vi "Fetch 5034B.vi"(8 "error in (no error)":errorcluster, 9 "MaxTime (10000ms)":u32=10000, 10 "Ch (1=Ch1)":u16(ring) items=["None", "Channel1", "Channel2", "Channel3", "Channel4", "Math1", "Math2", "Math3", "Math3", "Reference1", "Reference2", "Reference3", "Reference4"], 11 "VISA resource name":refnum<visa-resource-name>) -> (0 "error out":errorcluster, 1 "Data Cluster":cluster{"Y":dbl[], "t0":dbl, "dt":dbl}, 2 "Waveform Data":waveform(dbl)(graph)={"t0"=timestamp(3.694502999999883e-07 s since 1904-01-01), "dt"=5e-07, "Y"=array[10000 elements]}, 3 "VISA ResNameOut":refnum<visa-resource-name>)   [LabVIEW 2012]
doc: "Returns the waveform that an oscilloscope acquires for a channel you specify. An acquisition that you initiate before calling this VI generates the waveform.\n\nYou first enable channels with the tkdpo7k Configure Channel VI. Then you use the tkdpo7k Initiate VI to start an acquisition on the enabled channels. An oscilloscope concurrently acquires waveforms for these channels. You must call the tkdpo7k Fetch Waveform VI separately to obtain waveforms for each enabled channel. However, you also can call the tkdpo7k Read Waveform VI instead of using the above low-level VIs.\n\n<B>Note:</B> Use the tkdpo7k Fetch Waveform VI only with other low-level VIs, such as the tkdpo7k Initiate VI, the tkdpo7k Abort VI, and the tkdpo7k Fetch Waveform Measurement VI. High-level VIs such as the tkdpo7k Read Waveform VI automatically incorporate the functions of the tkdpo7k Initiate VI and the tkdpo7kFetch Waveform VI. The tkdpo7k Fetch Waveform VI does not check the status of an instrument."
panel:
  out "Data5064":dbl[](array[numeric])
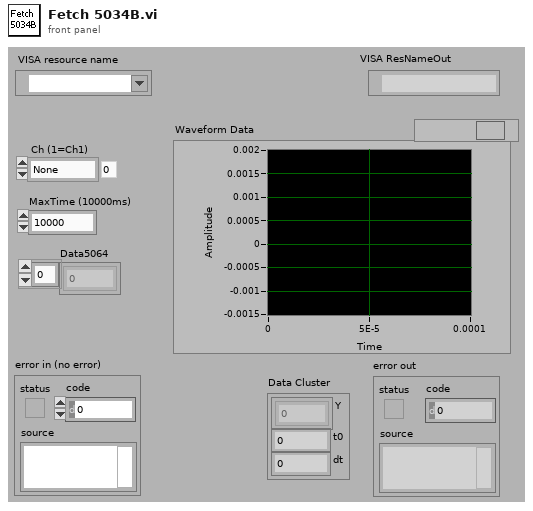
[diagram p1: front panel]
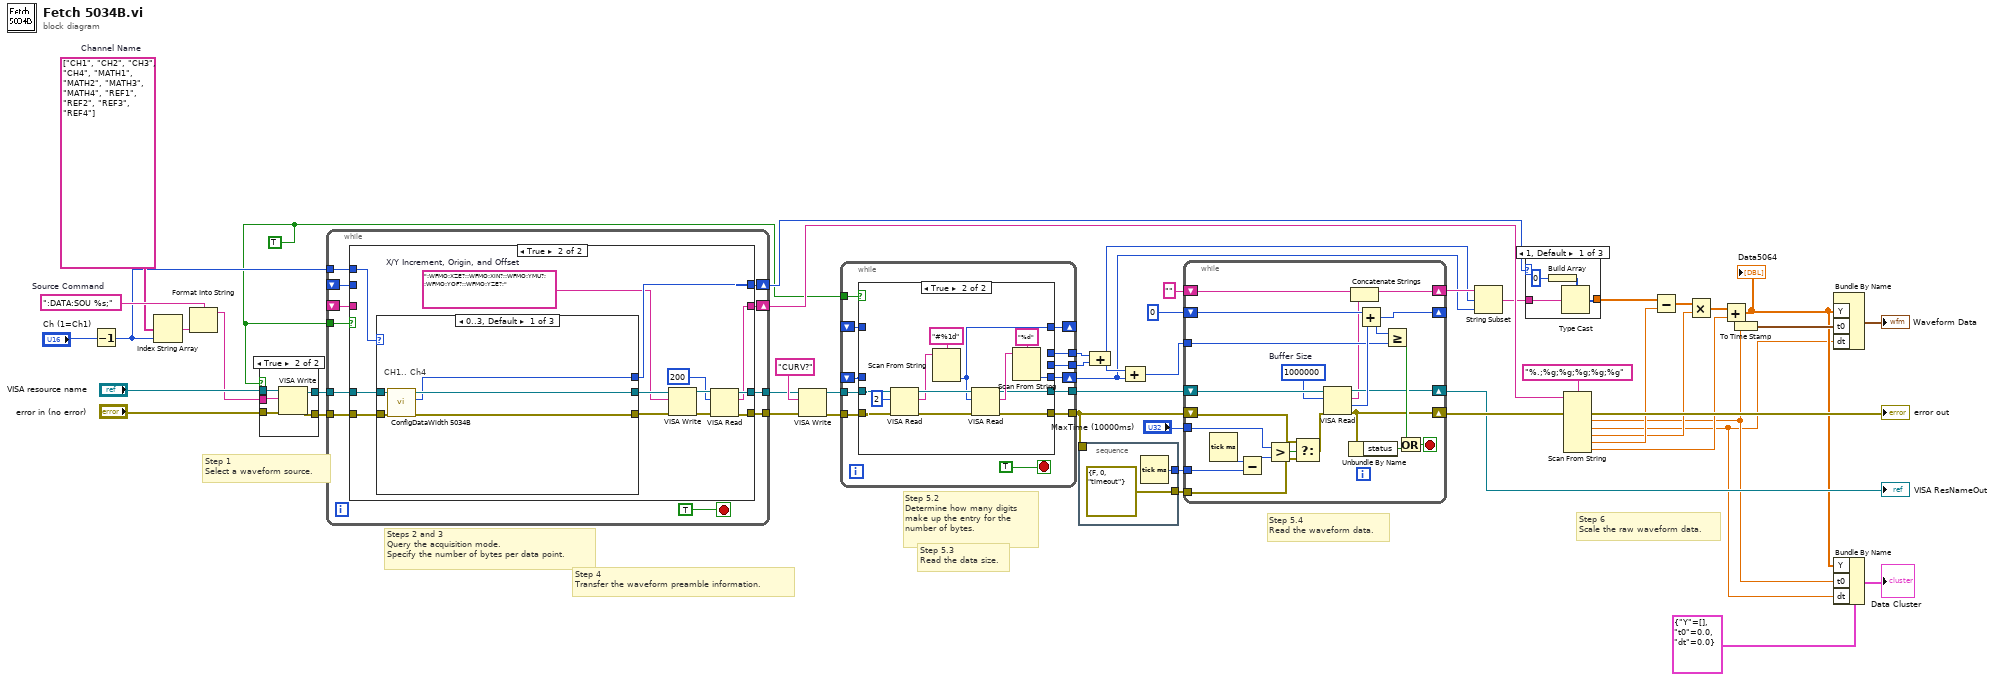
[diagram p0: block diagram]
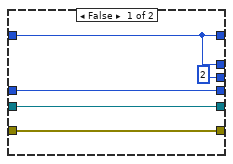
[diagram p3: hidden frame]
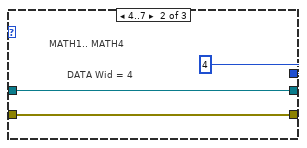
[diagram p5: hidden frame]
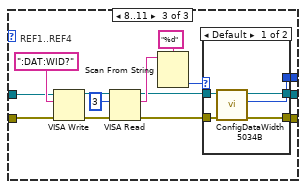
[diagram p6: hidden frame]
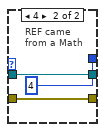
[diagram p7: hidden frame]
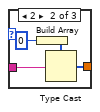
[diagram p8: hidden frame]
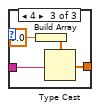
[diagram p9: hidden frame]
diagram:
  w6 = TRUE
  w37 = string[] ["CH1", "CH2", "CH3", "CH4", "MATH1", "MATH2", "MATH3", "MATH4", "REF1", "REF2", "REF3", "REF4"]  # Channel Name
  w49 = ":DATA:SOU %s;"  # Source Command
  # "Step 1       \nSelect a waveform source."
  # "Steps 2 and 3\nQuery the acquisition mode. \nSpecify the number of bytes per data point."
  # "Step 6    \nScale the raw waveform data."
  # "Step 5.4   \nRead the waveform data."
  # "Step 5.3      \nRead the data size."
  # "Step 5.2      \nDetermine how many digits\nmake up the entry for the \nnumber of bytes."
  # "Step 4\nTransfer the waveform preamble information."
  n1 = Decrement(x="Ch (1=Ch1)") -> (x-1=w7:u16)
  n2 = Index String Array(1:w7, 2:w37) -> (0:w48:string)  [unwired: 1 in]
  n3 = Format Into String(format string=w49, w48) -> (resulting string=w34:string)  [unwired: 2 in, 1 out]
  n4 = case shown="True" w6 {
    tunnel: "VISA resource name" -> [w51 w56]
    tunnel: "error in (no error)" -> [w50 w55]
    tunnel: w34 -> [_ w54]
    tunnel: [w51 w53] -> w31
    tunnel: [w50 w52] -> w30
    frame False {
    }
    frame True {
      n5 = VISA Write(VISA resource name=w56, write buffer=w54, error in (no error)=w55) -> (VISA resource name out=w53:refnum<visa-resource-name>, error out=w52:errorcluster)  [unwired: 1 out]
    }
  }
  n6 = while {
    tunnel: w7 -> [w67]
    tunnel: w31 -> [w66]
    tunnel: w30 -> [w65]
    tunnel: [w63] -> w21
    tunnel: [w62] -> w20
    tunnel: w6 -> [w61]
    shift-right: [w64] -> w23
    shift-left: _ -> [w59]
    shift-right: [w58] -> w22
    shift-left: _ -> [w57]
    stop <- TRUE stop-if-true
    n7 = case shown="True" w61 {
      tunnel: w67 -> [_ w84]
      tunnel: w66 -> [w71 w83]
      tunnel: w65 -> [w70 w82]
      tunnel: [w69 w81] -> w64
      tunnel: [w71 w75] -> w63
      tunnel: [w70 w74] -> w62
      tunnel: w59 -> [w69 _]
      tunnel: [w68 w72] -> w58
      tunnel: w57 -> [w68 _]
      frame False {
      }
      frame True {
        w73 = ":WFMO:XZE?;:WFMO:XIN?;:WFMO:YMU?;:WFMO:YOF?;:WFMO:YZE?;"  # X/Y Increment, Origin, and Offset
        n8 = case shown="0..3, Default" w84 {
          tunnel: w83 -> [w89 w92 w101]
          tunnel: w82 -> [w88 w91 w102]
          tunnel: [w87 w92 w95] -> w77
          tunnel: [w86 w91 w94] -> w76
          tunnel: [w85 u32 4 ("byte count") w93] -> w81
          frame 0..3, Default {
            # "CH1.. Ch4"
            n9 = call "ConfigDataWidth 5034B.vi"("error in (no error)"=w88, "VISA resource name"=w89) -> ("error out"=w86:errorcluster, "Width"=w85:i32, "VISA res name out"=w87:refnum<visa-resource-name>)  [unwired: 7 in]
          }
          frame 4..7 {
            # "DATA Wid = 4"
            # "MATH1.. MATH4"
          }
          frame 8..11 {
            # "REF1..REF4"
            n10 = VISA Write(VISA resource name=w101, write buffer=":DAT:WID?", error in (no error)=w102) -> (VISA resource name out=w106:refnum<visa-resource-name>, error out=w105:errorcluster)  [unwired: 1 out]
            n11 = VISA Read(VISA resource name=w106, byte count=u32 3, error in (no error)=w105) -> (VISA resource name out=w97:refnum<visa-resource-name>, read buffer=w100:string, error out=w96:errorcluster)  [unwired: 1 out]
            n12 = Scan From String(format string="%d", input string=w100) -> (output 1=w98:i32)  [unwired: 3 in, 3 out]
            n13 = case shown="Default" w98 {
              tunnel: w97 -> [w111 w114]
              tunnel: w96 -> [w110 w113]
              tunnel: [w109 w114] -> w95
              tunnel: [w108 w113] -> w94
              tunnel: [w107 u32 4 ("byte count")] -> w93
              frame Default {
                n14 = call "ConfigDataWidth 5034B.vi"("error in (no error)"=w110, "VISA resource name"=w111) -> ("error out"=w108:errorcluster, "Width"=w107:i32, "VISA res name out"=w109:refnum<visa-resource-name>)  [unwired: 7 in]
              }
              frame 4 {
                # "REF came\nfrom a Math"
              }
            }
          }
        }
        n15 = VISA Write(VISA resource name=w77, write buffer=w73, error in (no error)=w76) -> (VISA resource name out=w79:refnum<visa-resource-name>, error out=w80:errorcluster)  [unwired: 1 out]
        n16 = VISA Read(VISA resource name=w79, byte count=u32 200, error in (no error)=w80) -> (VISA resource name out=w75:refnum<visa-resource-name>, read buffer=w72:string, error out=w74:errorcluster)  [unwired: 1 out]
      }
    }
  }
  n17 = VISA Write(VISA resource name=w21, write buffer="CURV?" ("Curve Command"), error in (no error)=w20) -> (VISA resource name out=w29:refnum<visa-resource-name>, error out=w46:errorcluster)  [unwired: 1 out]
  n18 = while {
    tunnel: w46 -> [w126]
    tunnel: w29 -> [w125]
    tunnel: [w124] -> w28
    tunnel: [w123] -> w9
    tunnel: w6 -> [w122]
    shift-right: [w120] -> w11
    shift-left: _ -> [w119]
    shift-right: [w116] -> _
    shift-left: _ -> [w118]
    tunnel: [w117] -> w14
    tunnel: [w115] -> w13
    stop <- TRUE stop-if-true
    n19 = case shown="True" w122 {
      tunnel: w126 -> [w129 w144]
      tunnel: w125 -> [w130 w137]
      tunnel: [w130 w136] -> w124
      tunnel: [w129 w135] -> w123
      tunnel: [w131 w133] -> w120
      tunnel: w119 -> [w131 _]
      tunnel: [w127 w132] -> w116
      tunnel: w118 -> [w127 _]
      tunnel: [u32 2 ("byte count") _] -> w117
      tunnel: [w127 _] -> w115
      frame False {
      }
      frame True {
        n20 = VISA Read(VISA resource name=w137, byte count=u32 2, error in (no error)=w144) -> (VISA resource name out=w142:refnum<visa-resource-name>, read buffer=w140:string, error out=w141:errorcluster)  [unwired: 1 out]
        n21 = Scan From String(format string="#%1d", input string=w140) -> (output 1=w132:i32)  [unwired: 3 in, 3 out]
        n22 = VISA Read(VISA resource name=w142, byte count=w132, error in (no error)=w141) -> (VISA resource name out=w136:refnum<visa-resource-name>, read buffer=w138:string, error out=w135:errorcluster)  [unwired: 1 out]
        n23 = Scan From String(format string="%d", input string=w138) -> (output 1=w133:i32)  [unwired: 3 in, 3 out]
      }
    }
  }
  n24 = stacked-sequence {
    tunnel: [w146] -> w25
    tunnel: [errorcluster {"status"=FALSE, "code"=0, "source"="timeout"} ("error out")] -> w19
    tunnel: w9 -> [_]
    frame #0 {
      n25 = Tick Count (ms)() -> (millisecond timer value=w146:u32)
    }
  }
  n26 = Compound Arithmetic op=ADD(w13, w14) -> (w12:u32)
  n27 = Compound Arithmetic op=ADD(w12, w11) -> (w15:u32)
  n28 = while {
    shift-right: [w151] -> w43
    shift-left: w28 -> [w168]
    shift-right: [w147] -> w45
    shift-left: w9 -> [w155]
    shift-right: [w148] -> w16
    shift-left: "" -> [w150]
    tunnel: w15 -> [w153]
    shift-right: [w165] -> _
    shift-left: u32 0 -> [w166]
    tunnel: w25 -> [w163]
    tunnel: "MaxTime (10000ms)" -> [w162]
    tunnel: w19 -> [w160]
    stop <- w158 stop-if-true
    w152 = 1000000  # Buffer Size
    n29 = Tick Count (ms)() -> (millisecond timer value=w164:u32)
    n30 = Subtract(x=w164, y=w163) -> (x-y=w161:u32)
    n31 = Greater?(x=w162, y=w161) -> (0:w154:bool)
    n32 = Select(t=w155, s=w154, f=w160) -> (s? t:f=w157:errorcluster)
    n33 = VISA Read(VISA resource name=w168, byte count=w152, error in (no error)=w157) -> (VISA resource name out=w151:refnum<visa-resource-name>, read buffer=w149:string, return count=w167:u32, error out=w147:errorcluster)
    n34 = Unbundle By Name(w147) -> ("status"=w156:bool)
    n35 = Concatenate Strings(w150, w149) -> (w148:string)
    n36 = Add(x=w166, y=w167) -> (x+y=w165:u32)
    n37 = Greater Or Equal?(x=w165, y=w153) -> (x >= y?=w159:bool)
    n38 = Or(x=w159, y=w156) -> (x .or. y?=w158:bool)
  }
  "VISA ResNameOut" <- w43
  n39 = String Subset(string=w16, offset (0)=w12, length (rest)=w11) -> (substring=w10:string)
  n40 = case shown="1, Default" w23 {
    tunnel: w10 -> [w170 w174 w178]
    tunnel: [w169 w173 w177] -> w32
    frame 1, Default {
      n41 = Build Array(i8 0) -> (w171:i8[])
      n42 = Type Cast(type=w171, x=w170) -> (*(type *) &x=w169:i8[])
    }
    frame 2 {
      n43 = Build Array(i16 0 ("element")) -> (w175:i16[])
      n44 = Type Cast(type=w175, x=w174) -> (*(type *) &x=w173:i16[])
    }
    frame 4 {
      n45 = Build Array(sgl 0.0 ("element")) -> (w179:sgl[])
      n46 = Type Cast(type=w179, x=w178) -> (*(type *) &x=w177:sgl[])
    }
  }
  n47 = Scan From String(format string="%.;%g;%g;%g;%g;%g", input string=w22, error in=w45) -> (error out=→"error out":errorcluster, output 1=w2:dbl, output 2=w1:dbl, output 3=w38:dbl, output 4=w39:dbl, output 5=w26:dbl)  [unwired: 6 in, 2 out]
  n48 = Subtract(x=w32, y=w39) -> (x-y=w40:dbl[])
  n49 = Multiply(x=w40, y=w38) -> (x*y=w27:dbl[])
  n50 = Add(x=w27, y=w26) -> (x+y=w3:dbl[])
  "Data5064" <- w3
  n51 = To Time Stamp(1:w2) -> (0:w18:timestamp)
  n52 = Bundle By Name ("Build Waveform")("Y"=w3, "t0"=w18, "dt"=w1) -> (→"Waveform Data":waveform(dbl))  [unwired: 1 in]
  n53 = Bundle By Name(cluster=cluster{"Y":dbl[], "t0":dbl, "dt":dbl} {"Y"=[], "t0"=0.0, "dt"=0.0} ("Data Cluster"), "Y"=w3, "t0"=w2, "dt"=w1) -> (→"Data Cluster":cluster{"Y":dbl[], "t0":dbl, "dt":dbl})
